vi "Get Refnum Type From TD.vi"(4 "Type Descriptor":T1) -> (1 "Refnum Subtype Enum":T2 format="%02x")   [LabVIEW 2012, in "TD Tools.lvlib"]
uses:
  TD Tools.lvlib
  Custom Type/Refnum Subtype Enum.ctl
  Custom Type/Type Descriptor.ctl
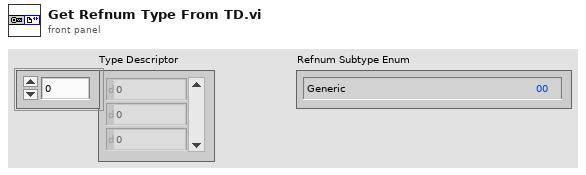
[diagram p1: front panel]
types:
  T1 = typedef "TD Tools.lvlib/Type Descriptor.ctl" = u16[]
  T2 = typedef "TD Tools.lvlib/Refnum Subtype Enum.ctl" = enum8{"Generic", "Datalog File Refnum", "Byte Stream File Refnum", "Device Refnum", "Occurence Refnum", "TCP Connection Refnum", "VISA Refnum (Obsolete)", "Automation Renum", "VI Server Refnum", "Menu Refnum", "IVI Refnum (Obsolete)", "IMAQ Session", "0x0C", "Datasocket Refnum", "VISA Resource", "IVI Logical Name", "UDP Connection Refnum", "Notifier Refnum", "Queue Refnum", "IrDA Refnum", "Hardware Plugin Refnum", "Hardware Plugin Tag Refnum", "DAQmx Refnum", "Event Registration Refnum", ".NET Refnum", "User Event Refnum", "0x1A", "Event Callback", "0x1C", "0x1D", "Only Used Internal to LabVIEW", "Bluetooth", "Data Value References", "RT FIFO", "TDM Streaming"}
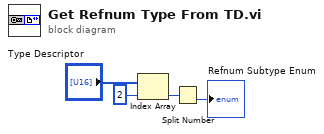
[diagram p0: block diagram]
diagram:
  n1 = Index Array(array="Type Descriptor", index=2 ("索引")) -> (element=w2:u16)
  n2 = Split Number(x=w2) -> (lo(x)=→"Refnum Subtype Enum":u8)  [unwired: 1 out]
